vi "Agilent VNA Convert Form 2 and 3 Numbers.vi"(4 "error in (no error)":errorcluster, 5 "data format (f)\n(f: Form 3; t: Form 2)":bool, 6 "input string":string) -> (0 "error out":errorcluster, 2 "Data":dbl[](array[numeric]) format="%.4e")   [LabVIEW 2011]
doc: "This VI for the HP8753B is used to convert form 2 and form 3 data arrays. Form 2 is IEEE 32-bit floating point format. Form 3 is IEEE 64-bit floating point format. Both formats are preceded by a 4-byte header which should be included with the \"input string\". As originally written, no VIs in the library use this VI. It is provided as a simple utility should anyone ever need it.\n\n This VI first pulls of the 4 byte header. The second pair of bytes could be converted to a 16-bit number to determine the length of the string which follows. This VI discards the header. \n\n The manuals say that form 2 numbers are 8 bytes and form 3 numbers are 16 bytes. This is because each number is really a pair of numbers. Each number in the pair must be converted separately. This VI is primarily a big loop. Each time through the loop, 4 or 8 bytes are pulled off the string and converted to a number which is then added to an array. Each number is converted with the \"Unflatten from String\" VI or with the \"Type Cast\" VI. For form2 numbers the type converted to should be \"single\"and for form3 numbers the type converted to should be \"double\". The loop executes until there is nothing left in the string."
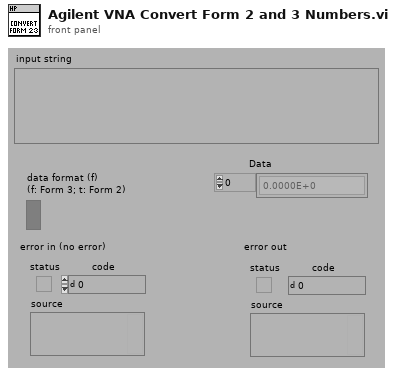
[diagram p1: front panel]
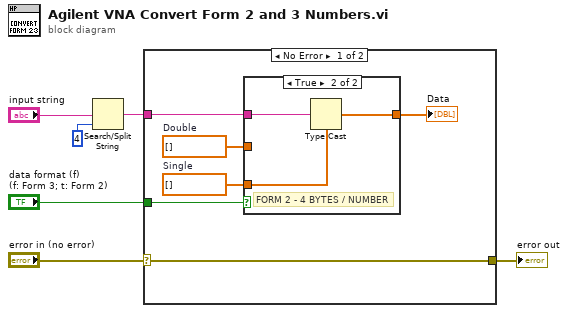
[diagram p0: block diagram]
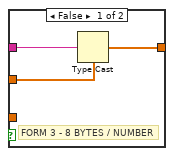
[diagram p2: hidden frame]
diagram:
  n1 = Search/Split String(string="input string", offset (0)=4) -> (match + rest of string=w4:string)  [unwired: 3 out]
  n2 = case shown="No Error" "error in (no error)" {
    selector: "error in (no error)" -> [w7 w19]
    tunnel: w4 -> [w11 _]
    tunnel: "data format (f)\n(f: Form 3; t: Form 2)" -> [w8 _]
    tunnel: [w7 w19] -> w1
    frame No Error {
      w10 = sgl[] []  # Single
      w9 = dbl[] []  # Double
      n3 = case shown="True" w8 {
        tunnel: w11 -> [w15 w18]
        tunnel: [w14 w17] -> w12
        tunnel: w9 -> [w13 _]
        tunnel: w10 -> [_ w16]
        frame False {
          # "FORM 3 - 8 BYTES / NUMBER"
          n4 = Type Cast(type=w13, x=w15) -> (*(type *) &x=w14:dbl[])
        }
        frame True {
          # "FORM 2 - 4 BYTES / NUMBER"
          n5 = Type Cast(type=w16, x=w18) -> (*(type *) &x=w17:sgl[])
        }
      }
      "Data" <- w12
    }
    frame Error {
    }
  }
  "error out" <- w1
